vi "String Compare Runtime Test.vi"() -> (0 "error out":errorcluster, 3 "Pass":bool)   [LabVIEW 2015, in "String Compare Tests.lvlib"]
uses:
  String Compare Tests.lvlib
  Config/String Compare Config.lvclass
  <vilib>/NI/Tag Bus/tag/Data Type.ctl
  <vilib>/NI/Tag Bus Module Framework/channel/channel classification.ctl
  classes/Step/Execution/StepState.ctl
  classes/Step/Execution/Step Status.ctl
  classes/Step/Execution/Step Flow Control.ctl
  Config/Mode.ctl
  Config/String Compare Config.lvclass/String Compare Config.ctl
  <vilib>/NI/Tag Bus/tag/tag descriptor.lvclass/tag descriptor.ctl
  <vilib>/NI/Tag Bus/table/data polymorphs/write one/write String.vi
  <vilib>/NI/Tag Bus/table/data polymorphs/read one/read Boolean.vi
  Config/Write Test Value Channel.vi
  Config/Write Result Channel.vi
  Config/Write Mode.vi
  Config/Write Limit_Regex.vi
  Config/Write ignore case.vi
  Config/Write Multiline.vi
  Config/Write offset.vi
  <vilib>/NI/Tag Bus/tag/read tag name.vi
  <vilib>/NI/Tag Bus/tag/read data type.vi
  <vilib>/NI/Tag Bus/dictionary/locate tag.vi
  classes/Step/Execution/Step.lvclass
  <vilib>/NI/Tag Bus Module Framework/channel/TBM channel.lvclass
  <vilib>/NI/Tag Bus/tag/tag descriptor.lvclass
  <vilib>/NI/Tag Bus/table/data table.lvlib
  <vilib>/NI/Tag Bus/dictionary/data dictionary.lvclass
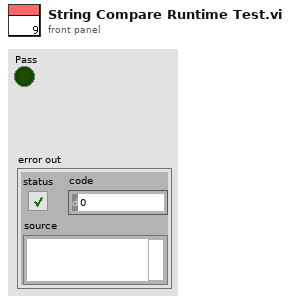
[diagram p1: front panel]
types:
  T1 = typedef "Step.lvclass/StepState.ctl" = cluster{"Step State":T2, "Flow Control":T3, "Jump Index":i32, "Done":bool}
  T2 = typedef "Step.lvclass/Step Status.ctl" = enum16{"Start", "Passed", "Failed", "Error", "Done", "Terminated", "Skipped", "Running"}
  T3 = typedef "Step.lvclass/Step Flow Control.ctl" = enum16{"Next Step", "Jump"}
  T4 = typedef "TBM channel.lvclass/channel classification.ctl" = enum16{"input data", "output data", "processing parameter", "processing result"}
  T5 = typedef "tag bus.lvlib/tag descriptor.lvclass/Data Type.ctl" = enum16{"Double", "Single", "I64", "I32", "I16", "I8", "U64", "U32", "U16", "U8", "Boolean", "String", "Array of Double", "Array of Single", "Array of I64", "Array of I32", "Array of I16", "Array of I8", "Array of U64", "Array of U32", "Array of U16", "Array of U8", "Array of Boolean", "Array of String"}
  T6 = typedef "String Compare Config.lvclass/Mode.ctl" = enum16{"Compare Strings", "Match Regex"}
  T7 = typedef "TBM channel.lvclass/data tables.ctl" = cluster{"input data":T8, "processing parameter":T8, "processing result":T8, "output data":T8}
  T8 = typedef "tag bus.lvlib/dictionary table pair.ctl" = cluster{"data dictionary":refnum<class "data dictionary.lvclass">, "data table":T9}
  T9 = typedef "tag bus.lvlib/data table.lvlib/data table.ctl" = cluster{"Double":dbl[], "Single":sgl[], "I64":i64[], "I32":i32[], "I16":i16[], "I8":i8[], "U64":u64[], "U32":u32[], "U16":u16[], "U8":u8[], "Boolean":bool[], "String":string[], "Array of Double":cluster{"DBL Array":dbl[]}[], "Array of Single":cluster{"SGL Array":sgl[]}[], "Array of I64":cluster{"I64 Array":i64[]}[], "Array of I32":cluster{"I32 Array":i32[]}[], "Array of I16":cluster{"I16 Array":i16[]}[], "Array of I8":cluster{"I8 Array":i8[]}[], "Array of U64":cluster{"U64 Array":u64[]}[], "Array of U32":cluster{"U32 Array":u32[]}[], "Array of U16":cluster{"U16 Array":u16[]}[], "Array of U8":cluster{"U8 Array":u8[]}[], "Array of Boolean":cluster{"Boolean Array":bool[]}[], "Array of String":cluster{"String Array":string[]}[]}
  T10 = cluster{"Step State":bool, "Flow Control":bool, "Jump Index":bool, "Done":bool}
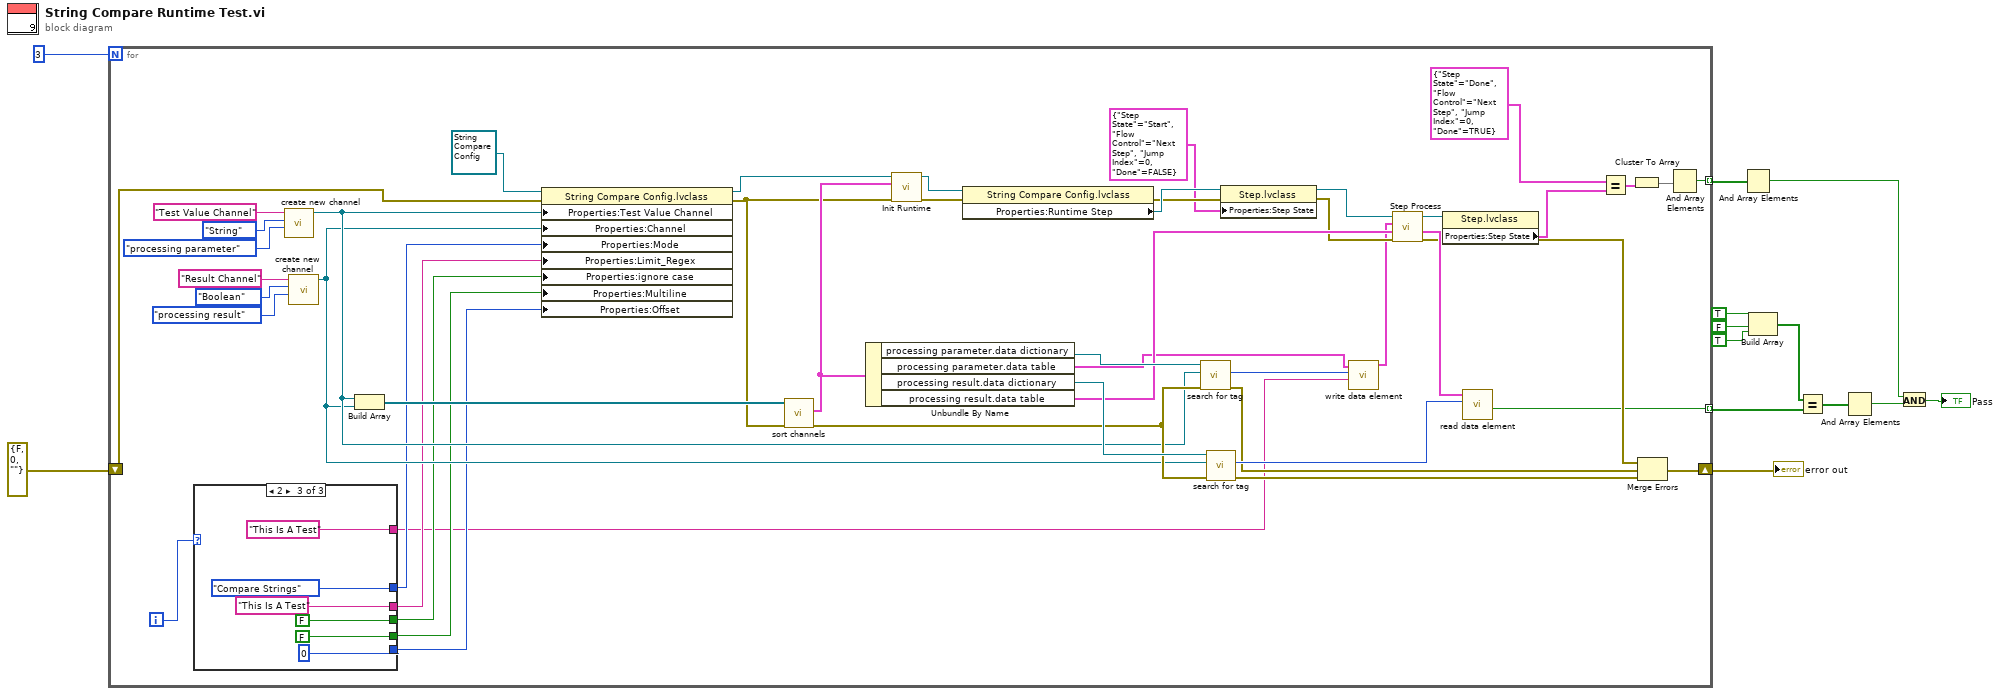
[diagram p0: block diagram]
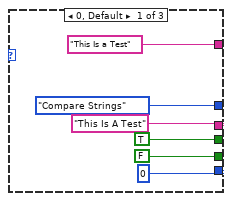
[diagram p2: hidden frame]
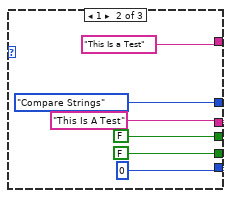
[diagram p3: hidden frame]
diagram:
  n1 = for {
    N: 3 -> [_]
    shift-right: [w38] -> w13
    shift-left: errorcluster {"status"=FALSE, "code"=0, "source"=""} ("error in (no error)") -> [w28]
    tunnel: [w20] -> w7 mode=indexing
    tunnel: [w16] -> w4 mode=indexing
    i -> [w27]
    n2 = case shown="2" w27 {
      tunnel: [Mode."Compare Strings" ("Mode") Mode."Compare Strings" ("Mode") Mode."Compare Strings" ("Mode")] -> w26
      tunnel: ["This Is A Test" ("Limit_Regex") "This Is A Test" ("Limit_Regex") "This Is A Test" ("Limit_Regex")] -> w25
      tunnel: [TRUE ("ignore case") FALSE ("ignore case") FALSE ("ignore case")] -> w24
      tunnel: [FALSE ("Multiline") FALSE ("Multiline") FALSE ("Multiline")] -> w23
      tunnel: [0 ("Offset") 0 ("Offset") 0 ("Offset")] -> w22
      tunnel: ["This Is a Test" ("Limit_Regex") "This Is a Test" ("Limit_Regex") "This Is A Test" ("Limit_Regex")] -> w21
      frame 0, Default {
      }
      frame 1 {
      }
      frame 2 {
      }
    }
    n3 = call <vilib>:"create new channel.vi"("channel classification"=channel_classification."processing parameter", "data type"=Data_Type."String", "channel name"="Test Value Channel") -> ("channel"=w32:refnum<class "TBM channel.lvclass">)  [unwired: 8 in]
    n4 = call <vilib>:"create new channel.vi"("channel classification"=channel_classification."processing result", "data type"=Data_Type."Boolean", "channel name"="Result Channel") -> ("channel"=w31:refnum<class "TBM channel.lvclass">)  [unwired: 8 in]
    n5 = Build Array(w32, w31) -> (w54:refnum<class "TBM channel.lvclass">[])
    n6 = property class="String Compare Config.lvclass"(reference=refnum<class "String Compare Config.lvclass"> refnum ("String Compare Config.lvclass"), error in=w28, "Properties:Test Value Channel"=w32, "Properties:Channel"=w31, "Properties:Mode"=w26, "Properties:Limit_Regex"=w25, "Properties:ignore case"=w24, "Properties:Multiline"=w23, "Properties:Offset"=w22) -> (reference out=w53:refnum<class "String Compare Config.lvclass">, error out=w37:errorcluster)
    n7 = call <vilib>:"sort channels.vi"("error in"=w37, "channels in"=w54) -> ("error out"=w42:errorcluster, "data allocations"=w52:T7)  [unwired: 7 in, 1 out]
    n8 = Unbundle By Name(w52) -> ("processing parameter.data dictionary"=w48:refnum<class "data dictionary.lvclass">, "processing parameter.data table"=w29:T9, "processing result.data dictionary"=w47:refnum<class "data dictionary.lvclass">, "processing result.data table"=w44:T9)
    n9 = call-dynamic "Init Runtime.vi"("error in (no error)"=w37, "data allocations"=w52, "String Compare Config in"=w53) -> ("error out"=w36:errorcluster, "String Compare Config out"=w51:refnum<class "String Compare Config.lvclass">)  [unwired: 6 in, 1 out]
    n10 = property class="String Compare Config.lvclass"(reference=w51, error in=w36) -> (error out=w41:errorcluster, "Properties:Runtime Step"=w50:refnum<class "Step.lvclass">)  [unwired: 1 out]
    n11 = call <vilib>:"search for tag.vi"("error in"=w42, "system tag"=w32, "data dictionary in"=w48) -> ("error out"=w40:errorcluster, "index"=w46:i32)  [unwired: 6 in, 1 out]
    n12 = call <vilib>:"search for tag.vi"("error in"=w42, "system tag"=w31, "data dictionary in"=w47) -> ("error out"=w39:errorcluster, "index"=w45:i32)  [unwired: 6 in, 1 out]
    n13 = property class="Step.lvclass"(reference=w50, error in=w41, "Properties:Step State"=T1 {"Step State"=enum."Start", "Flow Control"=enum."Next Step", "Jump Index"=0, "Done"=FALSE} ("Step State")) -> (reference out=w49:refnum<class "Step.lvclass">, error out=w35:errorcluster)
    n14 = call-poly <vilib>:"write data element.vi"("value"=w21, "index"=w46, "data table in"=w29) -> ("data table out"=w30:T9)  [unwired: 8 in]
    n15 = call-dynamic "Step Process.vi"("error in (no error)"=w35, "result allocation"=w44, "parameters"=w30, "Step in"=w49) -> ("error out"=w33:errorcluster, "results"=w43:T9, "Step out"=w15:refnum<class "Step.lvclass">)  [unwired: 4 in, 1 out]
    n16 = property class="Step.lvclass"(reference=w15) -> ("Properties:Step State"=w14:T1)  [unwired: 1 in, 2 out]
    n17 = call-poly <vilib>:"read data element.vi"("index"=w45, "data table in"=w43) -> ("value"=w20:bool)  [unwired: 8 in, 1 out]
    n18 = Equal?(x=T1 {"Step State"=enum."Done", "Flow Control"=enum."Next Step", "Jump Index"=0, "Done"=TRUE}, y=w14) -> (x = y?=w18:T10)
    n19 = Cluster To Array(cluster=w18) -> (array=w17:bool[])
    n20 = Merge Errors(w33, w40, w39) -> (w38:errorcluster)
    n21 = And Array Elements(Boolean array=w17) -> (logical AND=w16:bool)
  }
  "error out" <- w13
  n22 = And Array Elements(Boolean array=w4) -> (logical AND=w2:bool)
  n23 = Build Array(TRUE ("Multiline"), FALSE ("Multiline"), TRUE ("Multiline")) -> (w8:bool[])
  n24 = Equal?(x=w8, y=w7) -> (x = y?=w5:bool[])
  n25 = And Array Elements(Boolean array=w5) -> (logical AND=w3:bool)
  n26 = And(x=w2, y=w3) -> (x .and. y?=→"Pass":bool)
